vi "PH_ImageCalibrator.getCamsOnNode.vi"(0 "i ref in":refnum<vi>, 5 "error in (no error)":errorcluster) -> (14 "i ref out":refnum<vi>, 16 "cams on node":string[](array[string]), 19 "error out":errorcluster)   [LabVIEW 2014, in "PH_ImageCalibrator.lvlib"]
uses:
  PH_ImageCalibrator.lvlib
  CSCore/CSSystem/CSSystemLib/CSSystemLib.lvlib
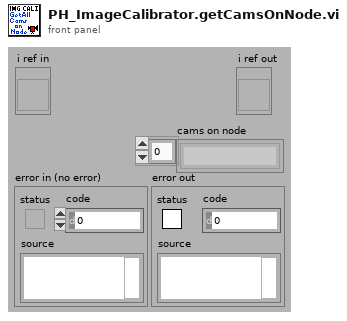
[diagram p1: front panel]
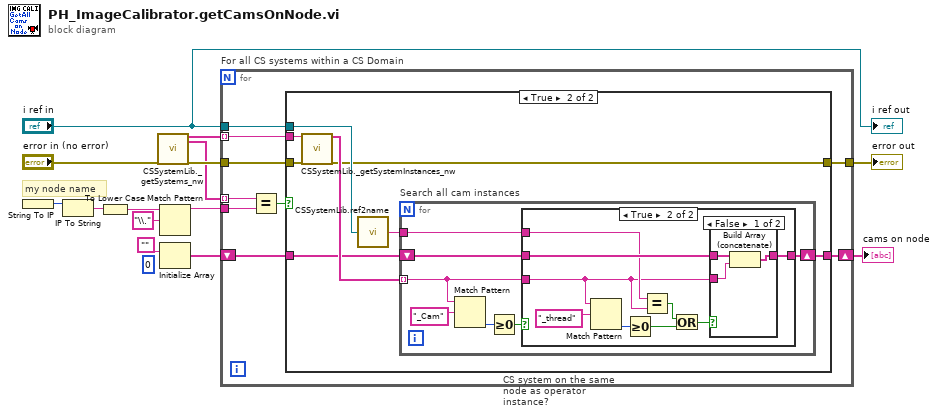
[diagram p0: block diagram]
diagram:
  (unwired) 0 ("dimension size")
  # "my node name"
  n1 = String To IP() -> (0:w10:u32)  [unwired: 1 in]
  n2 = IP To String(2:w10) -> (0:w9:string)  [unwired: 1 in]
  n3 = To Lower Case(string=w9) -> (all lower case string=w3:string)
  n4 = call "CSSystemLib._getSystems_nw.vi"("error in (no error)"="error in (no error)") -> ("CSSystems"=w12:string[], "CSNodes"=w8:string[], "error out"=w13:errorcluster)  [unwired: 16 in]
  n5 = Match Pattern(string=w3, regular expression="\\.") -> (before substring=w1:string)  [unwired: 1 in, 3 out]
  n6 = Initialize Array("") -> (w6:string[])  [unwired: 1 in]
  n7 = for "For all CS systems within a CS Domain" {
    tunnel: w13 -> [w23]
    tunnel: w12 -> [w22] mode=indexing
    tunnel: "i ref in" -> [w21]
    tunnel: w1 -> [w19]
    tunnel: w8 -> [w18] mode=indexing
    shift-right: [w16] -> w4
    shift-left: w6 -> [w17]
    tunnel: [w15] -> w5
    n8 = Equal?(x=w18, y=w19) -> (x = y?=w20:bool)
    n9 = case "CS system on the same node as operator instance?" shown="True" w20 {
      tunnel: w23 -> [w24 w33]
      tunnel: w22 -> [_ w32]
      tunnel: w21 -> [_ w29]
      tunnel: w17 -> [w25 w28]
      tunnel: [w25 w27] -> w16
      tunnel: [w24 w26] -> w15
      frame False {
      }
      frame True {
        n10 = call "CSSystemLib._getSystemInstances_nw.vi"("systemName"=w32, "error in (no error)"=w33) -> ("i list"=w31:string[], "error out"=w26:errorcluster)  [unwired: 16 in]
        n11 = call "CSSystemLib.ref2name.vi"("obj refnum"=w29) -> ("name"=w30:string)
        n12 = for "Search all cam instances" {
          shift-right: [w39] -> w27
          shift-left: w28 -> [w40]
          tunnel: w31 -> [w35] mode=indexing
          tunnel: w30 -> [w34]
          n13 = Match Pattern(string=w35, regular expression="_Cam") -> (offset past match=w37:i32)  [unwired: 1 in, 3 out]
          n14 = Greater Or Equal To 0?(x=w37) -> (x >= 0?=w36:bool)
          n15 = case shown="True" w36 {
            tunnel: w40 -> [w41 w50]
            tunnel: [w41 w49] -> w39
            tunnel: w35 -> [_ w43]
            tunnel: w34 -> [_ w46]
            frame False {
            }
            frame True {
              n16 = Match Pattern(string=w43, regular expression="_thread") -> (offset past match=w47:i32)  [unwired: 1 in, 3 out]
              n17 = Greater Or Equal To 0?(x=w47) -> (x >= 0?=w45:bool)
              n18 = Equal?(x=w46, y=w43) -> (x = y?=w42:bool)
              n19 = Or(x=w42, y=w45) -> (x .or. y?=w44:bool)
              n20 = case shown="False" w44 {
                tunnel: w50 -> [w53 w54]
                tunnel: [w52 w54] -> w49
                tunnel: w43 -> [w51 _]
                frame False {
                  n21 = Build Array (concatenate)(w53, w51) -> (w52:string[])
                }
                frame True {
                }
              }
            }
          }
        }
      }
    }
  }
  "error out" <- w5
  "cams on node" <- w4
  "i ref out" <- "i ref in"
